vi "Get Target Type.vi"(7 "error in (no error)":errorcluster, 10 "node ref in":refnum<data-value>) -> (0 "error out":errorcluster, 2 "Target Type":T1, 3 "node ref out":refnum<data-value>)   [LabVIEW 2013, in "TDMS datalogger editor node.lvclass"]
uses:
  TDMS datalogger editor node.lvclass
  <vilib>/NI/Configuration Framework/Node/NISE_CEF_Node.lvclass
  <vilib>/NI/Tag Bus Module Framework/root configuration/Target Types.ctl
  <vilib>/NI/DCAF/Tag Editor Core/Configuration Editor/Classes/Targets/Targets.lvclass
  <vilib>/NI/DCAF/Tag Editor Core/Framework Configuration Classes/target configuration/PL_Target Configuration.lvclass/PL_Target Configuration.ctl
  <vilib>/NI/Configuration Framework/Node/NISE_CEF_Node.lvclass/NISE_CEF_Node.ctl
  <vilib>/NI/Configuration Framework/Node/ReadParent.vi
  <vilib>/NI/DCAF/Tag Editor Core/Framework Configuration Classes/target configuration/PL_Target Configuration.lvclass
  <vilib>/NI/Tag Bus Module Framework/root configuration/TBM configuration.lvclass
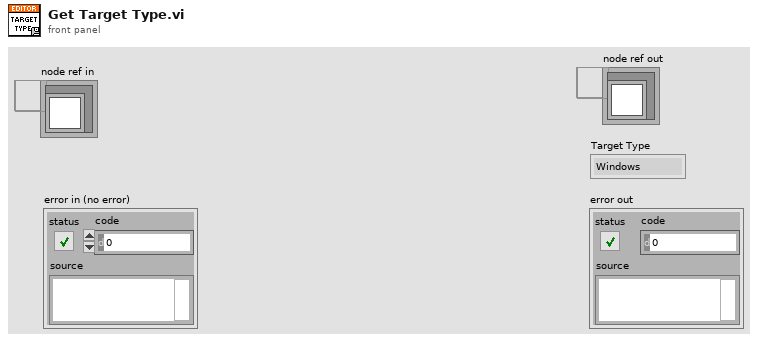
[diagram p1: front panel]
types:
  T1 = typedef "TBM configuration.lvclass/Target Types.ctl" = enum16{"Windows", "Mac", "Linux", "Linux RT ARM", "VxWorks", "Pharlap", "Other", "Linux RT x64"}
  T2 = typedef "NISE_CEF_Node.lvclass/NodeRef.ctl" = refnum<data-value>
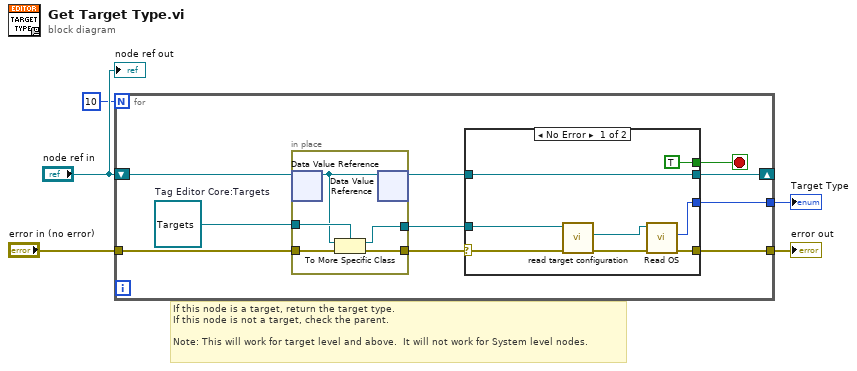
[diagram p0: block diagram]
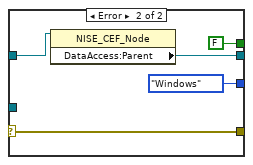
[diagram p2: hidden frame]
diagram:
  # "If this node is a target, return the target type.\nIf this node is not a target, check the parent.\n\nNote: This will work for target level and above.  It will not work for System level nodes."
  n1 = for {
    N: 10 -> [_]
    tunnel: [w10] -> w4
    shift-right: [w8] -> _
    shift-left: "node ref in" -> [w15]
    tunnel: "error in (no error)" -> [w7]
    tunnel: [w6] -> w1
    stop <- w12 stop-if-true
    w14 = refnum<class "Targets.lvclass"> refnum  # Tag Editor Core:Targets
    n2 = in-place {
      in-place-border: w14 -> [w33]
      in-place-border: [w32] -> w11
      in-place-border: [w31] -> w13
      in-place-border: w7 -> [w29]
      n3 = in-place-dvr #1(w15) -> (w30:refnum<class "NISE_CEF_Node.lvclass">)  [unwired: 1 out]
      n4 = To More Specific Class(target class=w33, reference=w30, error in=w29) -> (specific class reference=w32:refnum<class "Targets.lvclass">, error out=w31:errorcluster)
      n5 = in-place-dvr #1(w30) -> (w9:T2)  [unwired: 1 out]
    }
    n6 = case shown="No Error" w13 {
      selector: w13 -> [w20 w24]
      tunnel: [TRUE FALSE] -> w12
      tunnel: w11 -> [w19 _]
      tunnel: [w18 Target_Types."Windows" ("Target Types")] -> w10
      tunnel: w9 -> [w17 w26]
      tunnel: [w17 w25] -> w8
      tunnel: [w16 w24] -> w6
      frame No Error {
        n7 = call <vilib>:"read target configuration.vi"("error in"=w20, "Targets in"=w19) -> ("error out"=w22:errorcluster, "Target Configuration"=w23:refnum<class "PL_Target Configuration.lvclass">)  [unwired: 7 in, 1 out]
        n8 = call <vilib>:"Read OS.vi"("error in"=w22, "PL_Target Configuration in"=w23) -> ("error out"=w16:errorcluster, "Target Types"=w18:T1)  [unwired: 7 in, 1 out]
      }
      frame Error {
        n9 = property class="NISE_CEF_Node"(reference=w26) -> ("DataAccess:Parent"=w25:T2)  [unwired: 1 in, 2 out]
      }
    }
  }
  "Target Type" <- w4
  "error out" <- w1
  "node ref out" <- "node ref in"
